vi "PDP Monitor.vi"(8 "error in":errorcluster) -> ()   [LabVIEW 2014]
uses:
  <vilib>/Platform/TimedLoop/XDataNode/timing_clust.ctl
  <vilib>/Platform/TimedLoop/XDataNode/nitl_modes.ctl
  <vilib>/Platform/TimedLoop/XDataNode/wakeup.ctl
  PDP Current TypeDef.ctl
  <vilib>/platform/TimedLoop/XDataNode/XDataNode.xnode
  <vilib>/Platform/TimedLoop/XDataNode/XDNodeRunTimeDep.lvlib
panel:
  out "PDP Currents Chart":T1(graph)
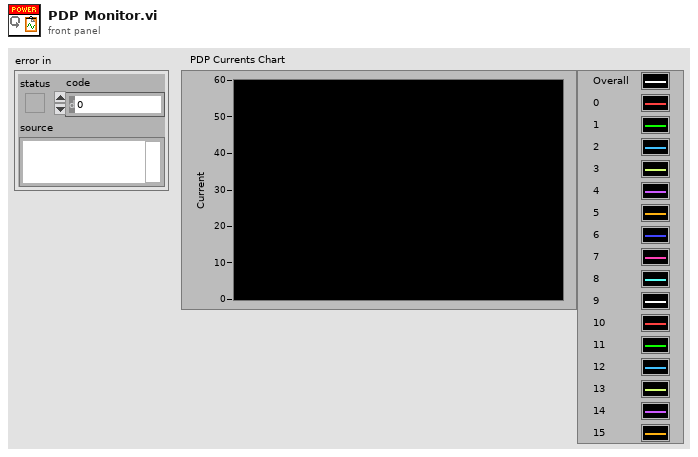
[diagram p1: front panel]
types:
  T1 = cluster{"Overall":dbl, "0":dbl, "1":dbl, "2":dbl, "3":dbl, "4":dbl, "5":dbl, "6":dbl, "7":dbl, "8":dbl, "9":dbl, "10":dbl, "11":dbl, "12":dbl, "13":dbl, "14":dbl, "15":dbl}
  T2 = enum16{"open", "replace", "create", "open or create", "replace or create", "replace or create with confirmation"}
  T3 = typedef "XDNodeRunTimeDep.lvlib/timing_clust.ctl" = cluster{"Expected End [f-1]":u64, "Actual End [f-1]":u64, "Finished Late? [f-1]":bool, "Expected End [i-1]":u64, "Actual End [i-1]":u64, "Finished Late? [i-1]":bool, "Expected Start [i]":u64, "Actual Start [i]":u64, "Expected Start [f]":u64, "Actual Start [f]":u64, "Source Name":string, "Structure Name":string, "Period":i64, "Deadline":i64, "Offset":i64, "Start":i64, "Priority":i32, "Timeout":i32, "Mode":T4, "Wakeup Reason":T5, "Error":errorcluster, "Source Type":string, "Secondary Source Type":string, "Global End Time":u64, "Global Start Time":u64, "Frame Duration":u64, "Iteration Duration":u64, "Assigned CPU":i32, "I/O Scan Engine Mode":u32}
  T4 = typedef "XDNodeRunTimeDep.lvlib/nitl_modes.ctl" = enum32{"No Change", "Process missed periods, maintain original phase", "Discard missed periods, maintain original phase", "Process missed periods, ignore original phase", "Discard missed periods, ignore original phase"}
  T5 = typedef "XDNodeRunTimeDep.lvlib/wakeup.ctl" = enum32{"Normal", "Aborted", "Asynchronous wakeup", "Timing source error", "Timed loop error", "Timeout"}
  T6 = typedef "PDP Current TypeDef.ctl" = cluster{"Overall":dbl, "0":dbl, "1":dbl, "2":dbl, "3":dbl, "4":dbl, "5":dbl, "6":dbl, "7":dbl, "8":dbl, "9":dbl, "10":dbl, "11":dbl, "12":dbl, "13":dbl, "14":dbl, "15":dbl}
  T7 = cluster{"[0]":dbl, "[1]":dbl, "[2]":dbl, "[3]":dbl, "[4]":dbl, "[5]":dbl, "[6]":dbl, "[7]":dbl, "[8]":dbl, "[9]":dbl, "[10]":dbl, "[11]":dbl, "[12]":dbl, "[13]":dbl, "[14]":dbl, "[15]":dbl, "[16]":dbl}
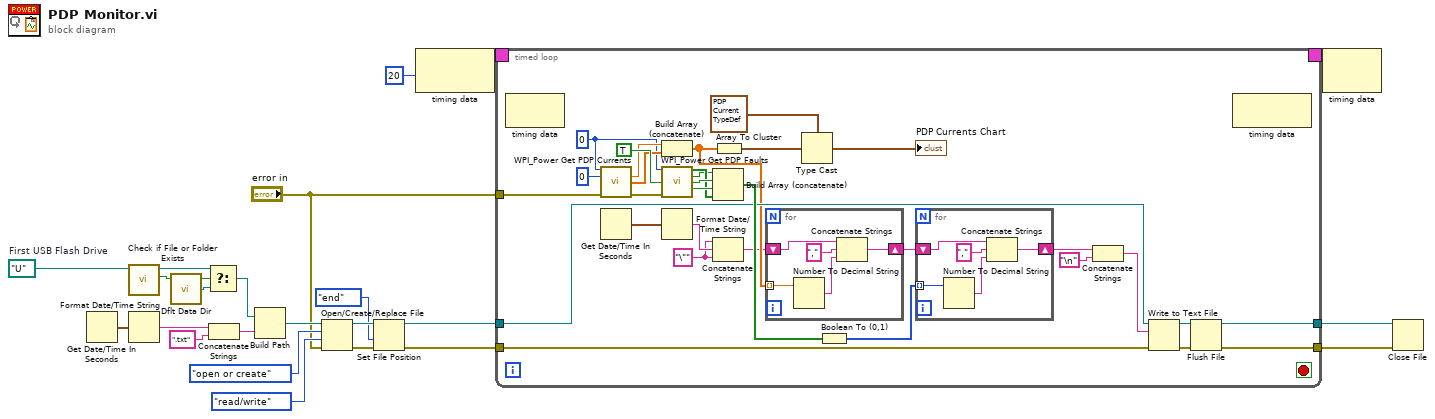
[diagram p0: block diagram]
diagram:
  w16 = path "U:/"  # First USB Flash Drive
  n1 = Get Date/Time In Seconds() -> (seconds since 1Jan1904=w9:timestamp)
  n2 = call <vilib>:"Check if File or Folder Exists.vi"("path"=w16) -> ("file or folder exists?"=w19:bool, "dup path"=w20:path)  [unwired: 8 in, 1 out]
  n3 = Format Date/Time String(seconds (now)=w9) -> (date/time string=w8:string)  [unwired: 2 in]
  n4 = call <vilib>:"Dflt Data Dir.vi"() -> ("App:Default Data Directory"=w18:path)
  n5 = Select(t=w20, s=w19, f=w18) -> (s? t:f=w17:path)
  n6 = Concatenate Strings(w8, ".txt" ("string")) -> (w7:string)
  n7 = Build Path(base path=w17, name or relative path=w7) -> (appended path=w15:path)
  n8 = Open/Create/Replace File(file path (use dialog)=w15, error in="error in", operation (0:open)=T2."open or create", access (0:read/write)=enum16{"read/write", "read-only", "write-only"}."read/write") -> (refnum out=w12:refnum<file>, error out=w11:errorcluster)  [unwired: 2 in, 1 out]
  n9 = Set File Position(refnum=w12, from (0:start)=enum16{"start", "end", "current"}."end", error in=w11) -> (refnum out=w5:refnum<file>, error out=w4:errorcluster)  [unwired: 1 in]
  n10 = node-c288(i64 20 ("Period")) -> (w23:T3)
  n11 = timed-loop {
    timing: w23 -> [_]
    timing-out: [_] -> w22
    tunnel: "error in" -> [w28]
    tunnel: w5 -> [w36]
    tunnel: w4 -> [w35]
    tunnel: [w30] -> w2
    tunnel: [w31] -> w3
    stop <- _ stop-if-true
    w25 = "\"" ("string")
    w47 = u8 0 ("Power Distribution Panel (0)")
    n12 = node-c288() -> ()  [unwired: 1 in, 1 out]
    n13 = call <vilib>:"WPI_Power Get PDP Currents.vi"("Power Distribution Panel (0)"=w47, "PDP Channel"=0, "error in"=w28) -> ("current (A)"=w52:dbl, "all currents (A)"=w51:dbl[], "error out"=w46:errorcluster)  [unwired: 10 in]
    n14 = Get Date/Time In Seconds() -> (seconds since 1Jan1904=w27:timestamp)
    n15 = Build Array (concatenate)(w52, w51) -> (w29:dbl[])
    n16 = call <vilib>:"WPI_Power Get PDP Faults.vi"("Power Distribution Panel (0)"=w47, "Clear Sticky Faults"=TRUE, "error in"=w46) -> ("Current Faults"=w43:bool[], "Battery Voltage Fault"=w42:bool, "Temperature Fault"=w45:bool, "Hardware Fault"=w44:bool)  [unwired: 8 in, 1 out]
    n17 = Format Date/Time String(seconds (now)=w27) -> (date/time string=w26:string)  [unwired: 2 in]
    n18 = Build Array (concatenate)(w42, w45, w44, w43) -> (w41:bool[])
    n19 = Concatenate Strings(w25, w26, w25) -> (w24:string)
    n20 = Array To Cluster(array=w29) -> (cluster=w50:T7)
    n21 = for {
      tunnel: w29 -> [w64] mode=indexing
      shift-right: [w60] -> w38
      shift-left: w24 -> [w63]
      n22 = Number To Decimal String(number=w64) -> (decimal integer string=w61:string)  [unwired: 1 in]
      n23 = Concatenate Strings(w63, "," ("string"), w61) -> (w60:string)
    }
    n24 = Type Cast(type=T6 {"Overall"=0.0, "0"=0.0, "1"=0.0, "2"=0.0, "3"=0.0, "4"=0.0, "5"=0.0, "6"=0.0, "7"=0.0, "8"=0.0, "9"=0.0, "10"=0.0, "11"=0.0, "12"=0.0, "13"=0.0, "14"=0.0, "15"=0.0} ("cluster"), x=w50) -> (*(type *) &x=→"PDP Currents Chart":T6)
    n25 = Boolean To (0,1)(Boolean=w41) -> (0, 1=w39:i16[])
    n26 = for {
      tunnel: w39 -> [w59] mode=indexing
      shift-right: [w55] -> w40
      shift-left: w38 -> [w58]
      n27 = Number To Decimal String(number=w59) -> (decimal integer string=w56:string)  [unwired: 1 in]
      n28 = Concatenate Strings(w58, "," ("string"), w56) -> (w55:string)
    }
    n29 = Concatenate Strings(w40, "\n") -> (w34:string)
    n30 = Write to Text File(file (use dialog)=w36, text=w34, error in=w35) -> (refnum out=w33:refnum<file>, error out=w32:errorcluster)  [unwired: 1 in, 1 out]
    n31 = Flush File(refnum=w33, error in=w32) -> (refnum out=w30:refnum<file>, error out=w31:errorcluster)
    n32 = node-c288() -> ()  [unwired: 1 in, 1 out]
  }
  n33 = node-c288(w22) -> ()  [unwired: 1 out]
  n34 = Close File(refnum=w2, error in=w3) -> ()  [unwired: 2 out]
